vi "Active_Power.vi"() -> ()   [LabVIEW 2015]
panel:
  out "Reactive Power":i32
  out "Active Power":i32
  out "Load Current":dynamicdata(graph)
  out "Voltage":dynamicdata(graph)
  out "Apparant Power":i32
  in  "Phase Difference":i32
  in  "Load Current":i32
  in  "Frequency":i32
  in  "Voltage":i32
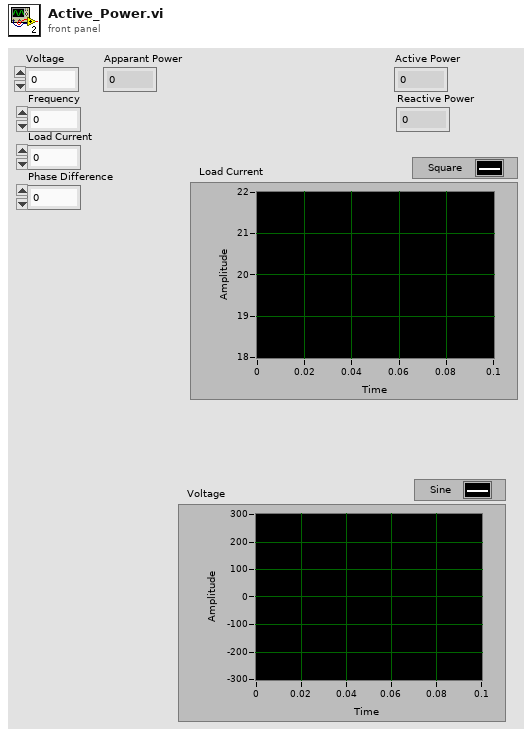
[diagram p1: front panel]
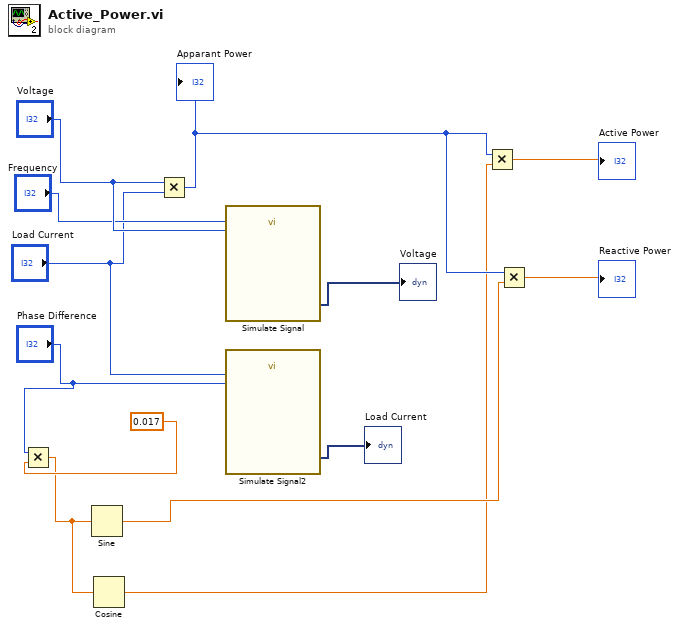
[diagram p0: block diagram]
diagram:
  n1 = Multiply(x="Phase Difference", y=0.017) -> (x*y=w1:dbl)
  n2 = Sine(x=w1) -> (sin(x)=w5:dbl)
  n3 = Cosine(x=w1) -> (cos(x)=w4:dbl)
  n4 = Multiply(x="Voltage", y="Load Current") -> (x*y=w8:i32)
  "Apparant Power" <- w8
  n5 = call "Simulate Signal"("Frequency"="Frequency", "Amplitude"="Voltage") -> ("Sine"=→"Voltage":dynamicdata)  [unwired: 12 in, 1 out]
  n6 = call "Simulate Signal2"("Amplitude"="Load Current", "Phase"="Phase Difference") -> ("Square"=→"Load Current":dynamicdata)  [unwired: 12 in, 1 out]
  n7 = Multiply(x=w8, y=w4) -> (x*y=→"Active Power":dbl)
  n8 = Multiply(x=w8, y=w5) -> (x*y=→"Reactive Power":dbl)
